vi "Close Connection.vi"(8 "error in (no error)":errorcluster, 11 "MB class in":refnum<class "MB class.lvclass">) -> (0 "error out":errorcluster, 3 "MB class out":refnum<class "MB class.lvclass">)   [LabVIEW 2020, in "MB class.lvclass"]
uses:
  MB class.lvclass
  MB class.lvclass/MB class.ctl
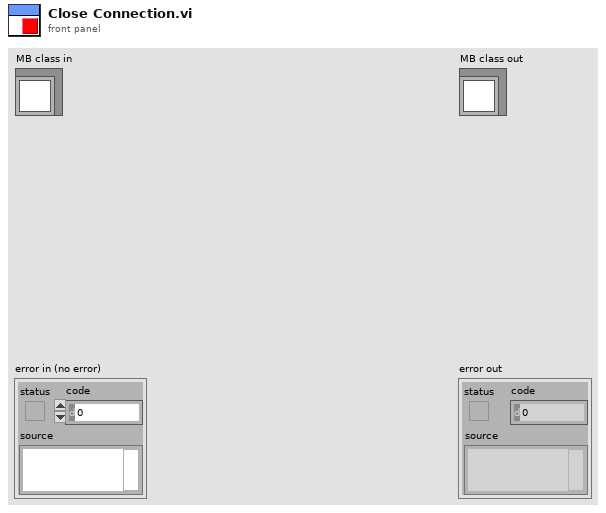
[diagram p1: front panel]
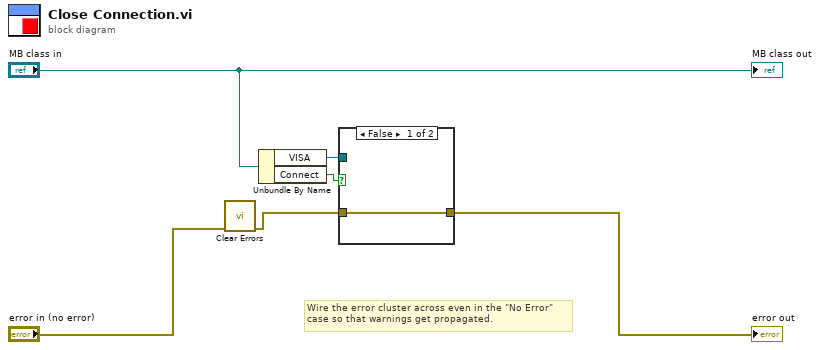
[diagram p0: block diagram]
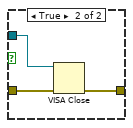
[diagram p2: hidden frame]
diagram:
  # "Wire the error cluster across even in the \"No Error\"\ncase so that warnings get propagated."
  n1 = call <vilib>:"Clear Errors.vi"("error in (no error)"="error in (no error)") -> ("error out"=w2:errorcluster)  [unwired: 5 in, 1 out]
  n2 = Unbundle By Name("MB class in") -> ("VISA"=w5:refnum<visa-resource-name>, "Connect"=w1:bool)
  n3 = case shown="False" w1 {
    tunnel: w5 -> [_ w10]
    tunnel: [w7 w9] -> w4
    tunnel: w2 -> [w7 w8]
    frame False {
    }
    frame True {
      n4 = VISA Close(VISA resource name=w10, error in (no error)=w8) -> (error out=w9:errorcluster)
    }
  }
  "error out" <- w4
  "MB class out" <- "MB class in"
